vi "To Variant.vi"(8 "error in":errorcluster, 11 "Boolean in":refnum<class "Path Builder.lvclass">) -> (0 "error out":errorcluster, 3 "Variant":variant)   [LabVIEW 2017, in "Custom Type Test Executive.lvlib" / "Path Builder.lvclass"]
uses:
  <vilib>/gpm_packages/@cs/test-executive/Source/Custom Type Test Executive/Path Builder Data Type/Path Builder.lvclass
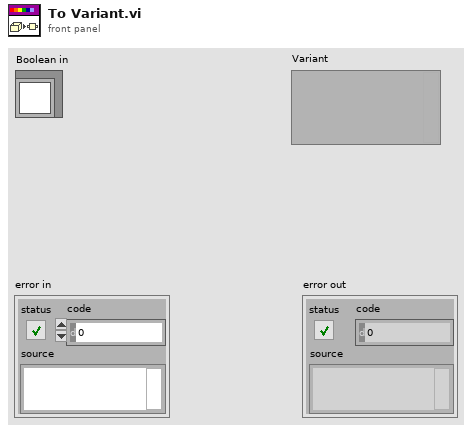
[diagram p1: front panel]
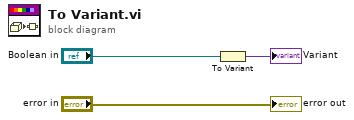
[diagram p0: block diagram]
diagram:
  n1 = To Variant(anything="Boolean in") -> (Variant=→"Variant":variant)
  "error out" <- "error in"
